vi "自动填充公式.vi"(7 "工作表名称":string="Sheet1", 8 "错误输入（无错误）":errorcluster, 11 "公式填充":T1 {"位置"."大小" min=1 max=1048576; "位置"."起始行" min=1 max=1048576; "填充区域"."大小" min=1 max=1048576; "填充区域"."起始行" min=1 max=1048576}) -> (0 "错误输出":errorcluster)   [LabVIEW 2020, in "OperateExcel.lvlib"]
uses:
  OperateExcel.lvlib
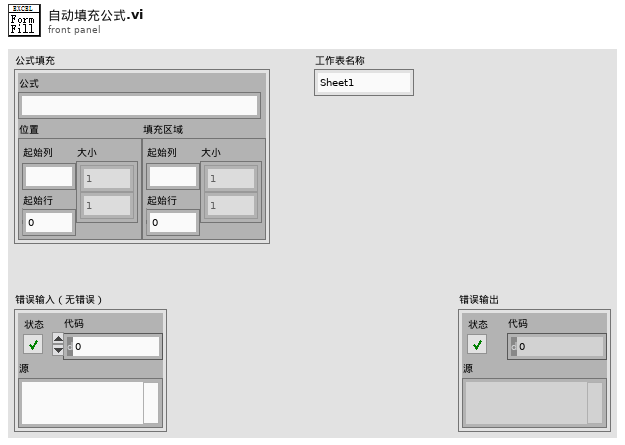
[diagram p1: front panel]
types:
  T1 = typedef "OperateExcel.lvlib/公式填充.ctl" = cluster{"公式":string, "位置":T2, "填充区域":T2}
  T2 = typedef "OperateExcel.lvlib/单元格区域.ctl" = cluster{"起始列":string, "起始行":u32, "大小":u32[]}
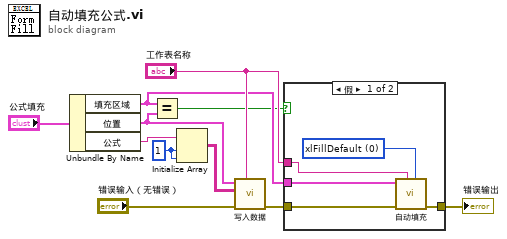
[diagram p0: block diagram]
diagram:
  w10 = 1 ("维数大小")
  n1 = Unbundle By Name("公式填充") -> ("填充区域"=w3:T2, "位置"=w2:T2, "公式"=w4:string)
  n2 = Equal?(x=w3, y=w2) -> (x = y?=w1:bool)
  n3 = Initialize Array(w4, w10, w10) -> (w9:string[][])
  n4 = call "写入数据.vi"("工作表名称"="工作表名称", "错误输入（无错误）"="错误输入（无错误）", "数据"=w9, "单元格区域"=w2) -> ("错误输出"=w8:errorcluster)  [unwired: 7 in]
  n5 = case shown="假" w1 {
    tunnel: w8 -> [w16 w17]
    tunnel: "工作表名称" -> [w15 _]
    tunnel: [w13 w17] -> w5
    tunnel: w3 -> [w12 _]
    frame False {
      w14 = 0 items=["xlFillCopy"=1, "xlFillDays"=5, "xlFillDefault"=0, "xlFillFormats"=3, "xlFillMonths"=7, "xlFillSeries"=2, "xlFillValues"=4, "xlFillWeekdays"=6, "xlFillYears"=8, "xlGrowthTrend"=10, "xlLinearTrend"=9, "xlFlashFill"=11] ("填充方式")
      n6 = call "自动填充.vi"("填充方式"=w14, "工作表名称"=w15, "错误输入（无错误）"=w16, "单元格区域"=w12) -> ("错误输出"=w13:errorcluster)  [unwired: 7 in]
    }
    frame True {
    }
  }
  "错误输出" <- w5
